vi "Close Topic Lookup Table Reference.vi"(8 "error in (no error)":errorcluster, 11 "TopicLookupTable":refnum<data-value>) -> (0 "error out":errorcluster)   [LabVIEW 2020, in "MVA Framework.lvlib" / "Mediator.lvlib" / "TopicLookupTable.lvclass"]
doc: "<License>\nCopyright © 2017 Composed Systems, LLC | All rights reserved\nwww.composed.io\n\nAuthor: Ethan Stern <ethan.stern@composed.io>\n\nThis software is provided \"AS IS\" WITHOUT WARRANTIES, either express or implied, AND IS FOR EDUCATIONAL PURPOSES ONLY.\n</License>"
uses:
  TopicLookupTable.lvclass
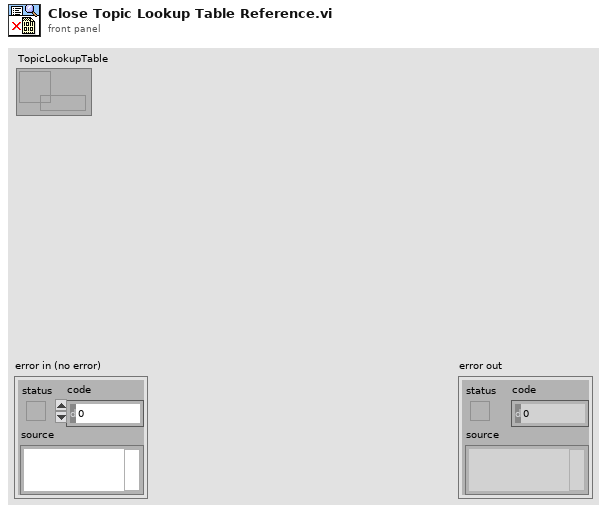
[diagram p1: front panel]
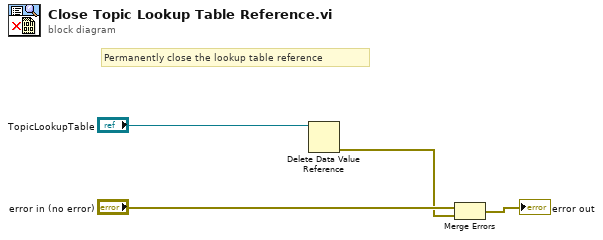
[diagram p0: block diagram]
diagram:
  # "Permanently close the lookup table reference"
  n1 = Delete Data Value Reference(data value reference="TopicLookupTable") -> (error out=w1:errorcluster)  [unwired: 1 in, 1 out]
  n2 = Merge Errors("error in (no error)", w1) -> (→"error out":errorcluster)
